vi "id.From JSON String.vi"(8 "error in (no error)":errorcluster, 10 "JSON String":string, 11 "id in":refnum<class "id.lvclass">) -> (0 "error out":errorcluster, 3 "id out":refnum<class "id.lvclass">)   [LabVIEW 2016, in "id.lvclass"]
uses:
  id.lvclass
  <vilib>/NI/JSON Support for LabVIEW/JSON Data Classes/JSON Datatype/JSON Null.lvclass
  <vilib>/NI/JSON Support for LabVIEW/JSON Data Classes/JSON Helper/Parsing/Parse Value.vi
  <vilib>/NI/JSON Support for LabVIEW/JSON Data Classes/JSON Helper/JSON Helper.lvclass
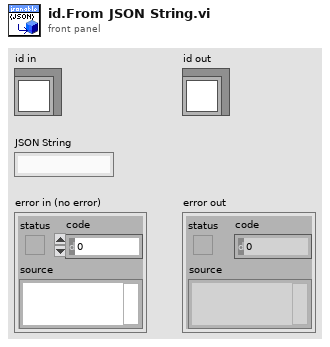
[diagram p1: front panel]
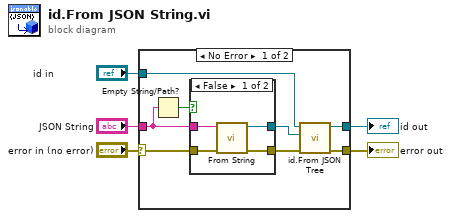
[diagram p0: block diagram]
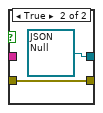
[diagram p2: hidden frame]
diagram:
  n1 = case shown="No Error" "error in (no error)" {
    selector: "error in (no error)" -> [w10 w21]
    tunnel: [w11 w21] -> w4
    tunnel: [w12 w20] -> w2
    tunnel: "id in" -> [w13 w20]
    tunnel: "JSON String" -> [w8 _]
    frame No Error {
      n2 = Empty String/Path?(string/path=w8) -> (empty?=w7:bool)
      n3 = case shown="False" w7 {
        tunnel: w8 -> [w17 _]
        tunnel: [w16 refnum<class "JSON Null.lvclass"> refnum ("JSON out")] -> w6
        tunnel: w10 -> [w14 w19]
        tunnel: [w15 w19] -> w9
        frame False {
          n4 = call <vilib>:"From String.vi"("error in (no error)"=w14, "JSON String"=w17) -> ("error out"=w15:errorcluster, "JSON out"=w16:refnum<class "JSON Null.lvclass">)  [unwired: 8 in]
        }
        frame True {
        }
      }
      n5 = call "id.From JSON Tree.vi"("error in (no error)"=w9, "JSON in"=w6, "id in"=w13) -> ("error out"=w11:errorcluster, "id out"=w12:refnum<class "id.lvclass">)  [unwired: 7 in]
    }
    frame Error {
    }
  }
  "error out" <- w4
  "id out" <- w2
